vi "NXT_DisplayText.vi"(7 "Clear Display (F)":bool, 9 "Text":string, 10 "Location (0,0)":cluster{"X":i16, "Y":i16}, 11 "Sequence Flow in":T2) -> (3 "Sequence Flow out":T2)   [LabVIEW 2009]
doc: "Writes a single line of text on the NXT display. Only characters that are supported by the NXT's built-in font will be displayed."
uses:
  <vilib>/NXT/NXT Controls/SequenceBoolean.ctl
  Library.llb/NXTSyscallRefnum.ctl
  C:/Program Files/National Instruments/LabVIEW 2009/resource/objmgr/NXTInputOutput.rc
panel:
  in  "Generic Refnum Name":T1
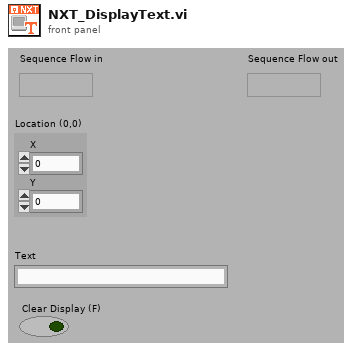
[diagram p1: front panel]
types:
  T1 = typedef "NXTSyscallRefnum.ctl" = refnum<k21>
  T2 = typedef "SequenceBoolean.ctl" = bool
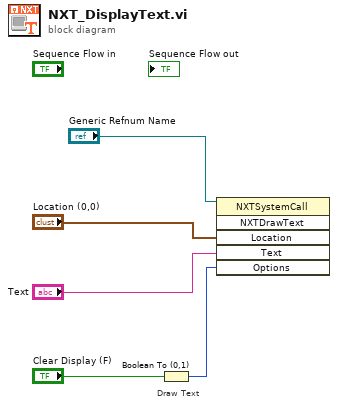
[diagram p0: block diagram]
diagram:
  # "Draw Text"
  n1 = Boolean To (0,1)(Boolean="Clear Display (F)") -> (0, 1=w2:i16)
  n2 = invoke class="NXTSystemCall" method="NXTDrawText"(reference="Generic Refnum Name", "Location"="Location (0,0)", "Text"="Text", "Options"=w2) -> ()  [unwired: 2 in, 6 out]
